vi "encoder_test_3mode_2motor_v4.vi"() -> ()   [LabVIEW 2014]
uses:
  <vilib>/rvi/FXPMathLib/FxpSinAndCos/subVIs/nifxpmath_SinAndCos_SimConfig.ctl
  <vilib>/rvi/Emulation/niFpgaGetClockAttributes.vi
  <vilib>/rvi/Emulation/niFpgaSctlEmulationGetInTimedLoop.vi
  <vilib>/rvi/Emulation/niFpgaEmulationReportErrorSimple.vi
  <vilib>/rvi/eio/common/nirviEmuTemplateMethod_errors.vi
  <vilib>/rvi/Emulation/niFpgaProcessEmulError.vi
  <vilib>/rvi/Emulation/niFpgaCriticalErrorInLSC.vi
  <vilib>/rvi/FXPMathLib/FxpSinAndCos/simVIs/DllFxpSinAndCosTemp_sub.vi
  <vilib>/rvi/interface/RandomDataEmulation/nirviRandomDataMultiElementFPGAFIFO.vi
  <instcachedir>/0/nirviRandomDataMultiElementFPGAFIFO_AD0CFC12EF974623A9C2E4184BC062B2.lvgen/nirviRandomDataMultiElementFPGAFIFO_AD0CFC12EF974623A9C2E4184BC062B2_020.vi
  <vilib>/rvi/interface/RandomDataEmulation/niFpgaRandomDataHandleErrors.vi
  <vilib>/eio/EIONode/EIONode.xnode
  <vilib>/rvi/FXPMathLib/FxpMul/XNode/nifxpmath_Multiplier.xnode
  <vilib>/rvi/FXPMathLib/FxpSinAndCos/XNode/nifxpmath_SinAndCos.xnode
  <vilib>/rvi/Analysis/measure/butterworth/XNode/niFpgaButterworthFilter.xnode
  <vilib>/rvi/FXPMathLib/FxpSub/XNode/nifxpmath_Sub.xnode
  <vilib>/rvi/FXPMathLib/FxpAdd/XNode/nifxpmath_Add.xnode
  <vilib>/rvi/DataTransferAndStorage/Container/XNode/niFpgaContainer.xnode
  <vilib>/rvi/interface/RandomDataEmulation/nirviRandomDataFpgaMultiElementTemplate.vi
  <vilib>/rvi/FXPMathLib/sim/FxpSim.dll
panel:
  in  "mt0_y":u32
  out "Dyr_sin_dd":fxp<+/-,64,25>
  out "Dyr_sin_d":fxp<+/-,64,16>
  out "Dyr_sin":fxp<+/-,30,11>
  in  "Sin offset_y":fxp<+/-,29,10>
  out "Sin omega_y":fxp<+/-,41,8>
  in  "Sin magnitude_y":fxp<+/-,11,8>
  in  "Sin frequency_y (Hz)":fxp<+/-,21,5>
  out "Dyr_ramp":fxp<+/-,32,7>
  out "Time now_y (s)":fxp<+,52,14>
  out "Dyr_slope":fxp<+/-,32,10>
  in  "Dyr_time":fxp<+/-,32,10>
  in  "Dyr_end":fxp<+/-,32,7>
  out "Dy_i":fxp<+/-,32,10>
  out "Dyr":fxp<+/-,32,7>
  in  "Direction_y":bool
  in  "Command type_y":i16(ring) items=["Step", "Ramp", "Sine"]
  out "Dy_error":fxp<+/-,24,8>
  out "Fmr_y":fxp<+/-,32,10>
  in  "Ki_y":fxp<+/-,20,6>
  in  "Dy_tolorence":fxp<+/-,18,1>
  in  "Kd_y":fxp<+/-,20,8>
  in  "Kp_y":fxp<+/-,20,8>
  in  "scaled coefficients_Dy_dd":i32[](array[numeric])=[780119100, 146811362]
  out "Dy_dd":fxp<+/-,36,10>
  out "va_y":fxp<+/-,38,8>
  out "vb_y":fxp<+/-,38,8>
  out "vd_y":fxp<+/-,20,5>
  out "vq_y":fxp<+/-,20,5> format="%.57g"
  in  "Stop motor_y":bool
  out "Dy_d (mm/s)":fxp<+/-,33,9>
  out "omega_y (rad/s)":fxp<+/-,32,7>
  in  "Velocity Estimation_y":i16(ring) items=["M_avg method", "M method", "T method"]
  out "Dy_d (T)":fxp<+/-,32,8>
  out "mt_y":u32
  out "omega_y (T)":fxp<+/-,32,7>
  out "omega_y (M)":fxp<+/-,32,7>
  out "Dy_d (M)":fxp<+/-,32,8>
  in  "Dy_d_M_Tc (mSec)":u32 format="%#_6f"
  out "omega_y(M_avg)":fxp<+/-,32,7>
  out "Dy_d (M_avg)":fxp<+,32,8>
  in  "Dy_d_M_avg_Tc (uSec)":u32
  out "rad_y(NrTheta)":fxp<+/-,33,18>
  out "Dy (mm)":fxp<+/-,22,7>
  out "Encoder Position_y":i32
  in  "Encoder Reset_y":bool
  out "omega_p (M_avg)":fxp<+/-,32,7>
  out "Dp_d (M_avg)":fxp<+/-,32,8>
  in  "Dp_d_M_avg_Tc (uSec)":u32 caption="D_d_M_avg_Tc (uSec)"
  out "omega_p (M)":fxp<+/-,32,7>
  out "Dp_d (M)":fxp<+/-,32,8>
  in  "Dp_d_M_Tc (mSec)":u32 format="%#_6f"
  out "Dp_d (T)":fxp<+/-,32,8>
  out "omega_p(T)":fxp<+/-,32,7>
  in  "Velocity Estimation_p":i16(ring) items=["M_avg method", "M method", "T method"]
  out "Dpr_ramp":fxp<+/-,64,30>
  out "Dpr_slope":fxp<+/-,32,10>
  in  "Dpr_time":fxp<+/-,32,10>
  out "Dpr_sin":fxp<+/-,30,11>
  out "Dpr_sin_d":fxp<+/-,64,16>
  out "Dpr_sin_dd":fxp<+/-,64,25>
  out "Sin omega_p":fxp<+/-,41,8>
  in  "Sin offset_p":fxp<+/-,27,10>
  in  "Sin magnitude_p":fxp<+/-,11,8>
  in  "Sin frequency_p (Hz)":fxp<+/-,21,5>
  out "Time now_p (s)":fxp<+,52,14>
  out "Dpr":fxp<+/-,32,7>
  in  "Dpr_end":fxp<+/-,22,7>
  in  "Command type_p":i16(ring) items=["Step", "Ramp", "Sine"]
  out "Dp_i":fxp<+/-,32,10>
  in  "Dp_tolorence":fxp<+/-,18,1>
  in  "Ki_p":fxp<+/-,20,6>
  out "Dp_error":fxp<+/-,24,8>
  in  "Direction_p":bool
  out "Fmr_p":fxp<+/-,32,10>
  in  "Kd_p":fxp<+/-,20,8>
  in  "Kp_p":fxp<+/-,20,12>
  in  "scaled coefficients_Dp_dd":i32[](array[numeric])=[780119100, 146811362]
  out "Dp_dd":fxp<+/-,36,10>
  in  "Ini coe.":bool
  out "va_p":fxp<+/-,38,8>
  out "vb_p":fxp<+/-,38,8>
  in  "Stop motor_p":bool
  out "vq_p":fxp<+/-,20,5> format="%.57g"
  out "vd_p":fxp<+/-,20,5>
  out "Dp_d (mm/s)":fxp<+/-,32,8>
  out "mt_p":u32
  out "omega_p (rad/s)":fxp<+/-,32,7>
  in  "mt0_p":u32
  out "Dp (mm)":fxp<+/-,22,7>
  out "rad_p(NrTheta)":fxp<+/-,33,18>
  out "Encoder Position_p":i32
  in  "Encoder Reset_p":bool
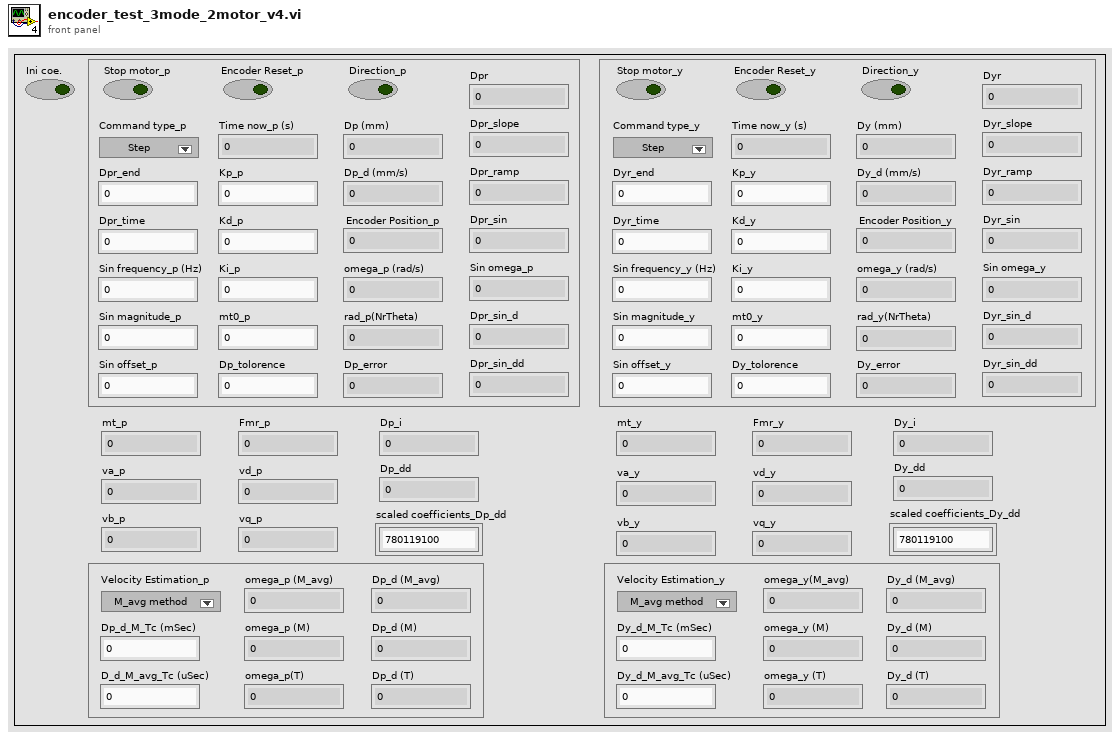
[diagram p1: front panel]
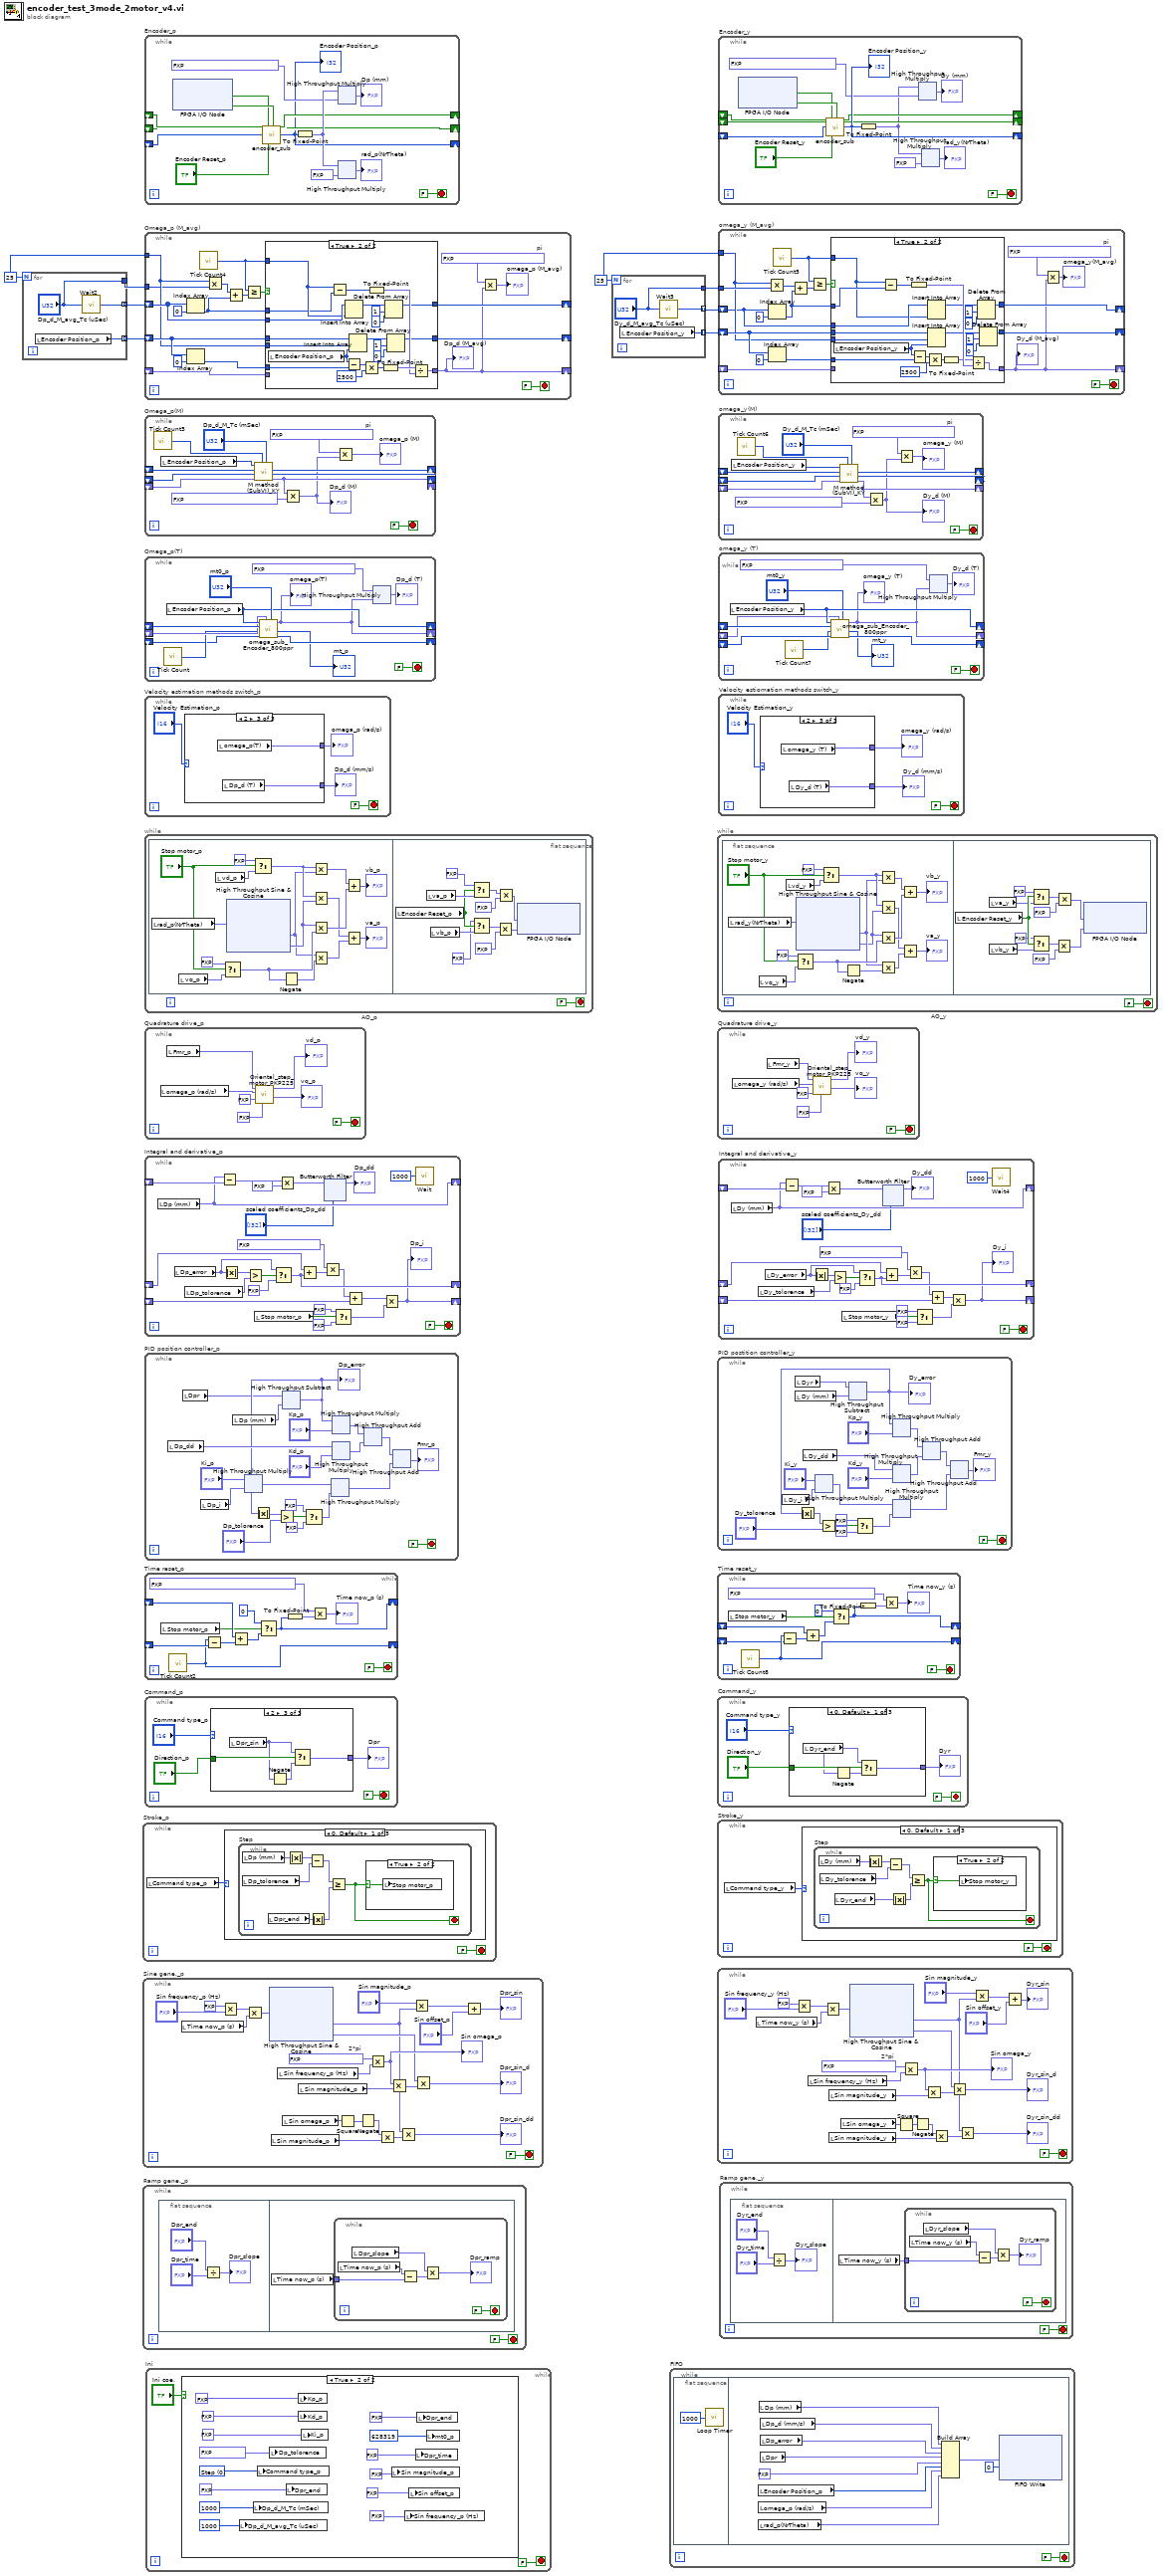
[diagram p0: block diagram]
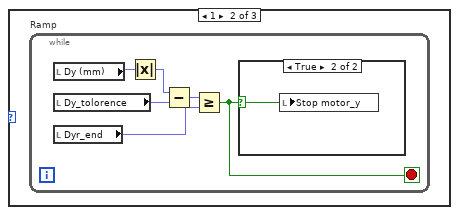
[diagram p3: hidden frame]
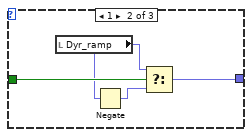
[diagram p6: hidden frame]
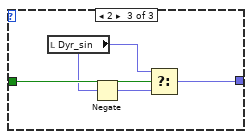
[diagram p7: hidden frame]
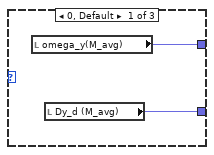
[diagram p8: hidden frame]
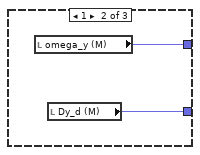
[diagram p9: hidden frame]
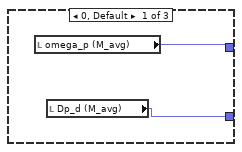
[diagram p12: hidden frame]
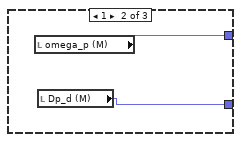
[diagram p13: hidden frame]
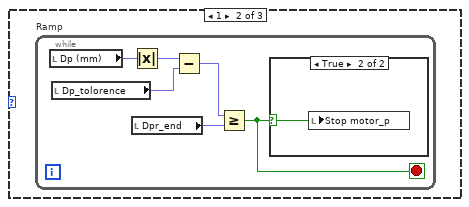
[diagram p15: hidden frame]
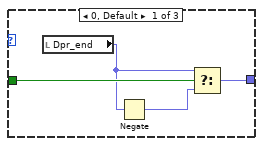
[diagram p18: hidden frame]
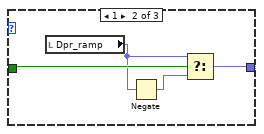
[diagram p19: hidden frame]
diagram:
  w4 = 25
  w8 = 25
  n1 = for {
    N: w8 -> [_]
    tunnel: ["Dp_d_M_avg_Tc (uSec)"] -> w5
    tunnel: [w10] -> w7 mode=indexing
    tunnel: [w9] -> w6 mode=indexing
    n2 = local read "Encoder Position_p"() -> (w9:i32)
    n3 = call "Wait2"("Count(uSec)"="Dp_d_M_avg_Tc (uSec)") -> ("Tick Count(uSec)"=w10:u32)
  }
  n4 = while "Stroke_p" {
    stop <- FALSE stop-if-true
    n5 = local read "Command type_p"() -> (w13:i16)
    n6 = case shown="0, Default" w13 {
      frame 0, Default {
        n7 = while "Step" {
          stop <- w14 stop-if-true
          n8 = local read "Dp_tolorence"() -> (w16:fxp<+/-,18,1>)
          n9 = local read "Dp (mm)"() -> (w18:fxp<+/-,22,7>)
          n10 = local read "Dpr_end"() -> (w20:fxp<+/-,22,7>)
          n11 = Absolute Value(x=w18) -> (abs(x)=w17:fxp<+,22,7>)
          n12 = Subtract(x=w17, y=w16) -> (x-y=w15:fxp<+/-,25,8>)
          n13 = Absolute Value(x=w20) -> (abs(x)=w19:fxp<+,22,7>)
          n14 = Greater Or Equal?(x=w15, y=w19) -> (x >= y?=w14:bool)
          n15 = case shown="True" w14 {
            selector: w14 -> [_ w21]
            frame False {
            }
            frame True {
              n16 = local write "Stop motor_p"(w21) -> ()
            }
          }
        }
      }
      frame 1 {
        n17 = while "Ramp" {
          stop <- w22 stop-if-true
          n18 = local read "Dp (mm)"() -> (w24:fxp<+/-,22,7>)
          n19 = local read "Dp_tolorence"() -> (w26:fxp<+/-,18,1>)
          n20 = Absolute Value(x=w24) -> (abs(x)=w25:fxp<+,22,7>)
          n21 = local read "Dpr_end"() -> (w23:fxp<+/-,22,7>)
          n22 = Subtract(x=w25, y=w26) -> (x-y=w27:fxp<+/-,25,8>)
          n23 = Greater Or Equal?(x=w27, y=w23) -> (x >= y?=w22:bool)
          n24 = case shown="True" w22 {
            selector: w22 -> [_ w28]
            frame False {
            }
            frame True {
              n25 = local write "Stop motor_p"(w28) -> ()
            }
          }
        }
      }
      frame 2 {
      }
    }
  }
  n26 = while "Sine gene._p" {
    stop <- FALSE stop-if-true
    w46 = fxp<+,20,3> 6.2831878662109375  # 2*pi
    n27 = local read "Time now_p (s)"() -> (w49:fxp<+,52,14>)
    n28 = Multiply(x=fxp<+,1,2> 2.0, y="Sin frequency_p (Hz)") -> (x*y=w50:fxp<+/-,21,6>)
    n29 = Multiply(x=w50, y=w49) -> (x*y=w30:fxp<+/-,64,20>)
    n30 = xnode "High Throughput Sine & Cosine"("x (pi)"=w30) -> ("sin(x)"=w34:fxp<+/-,18,2>, "cos(x)"=w41:fxp<+/-,18,2>)
    n31 = local read "Sin magnitude_p"() -> (w36:fxp<+/-,11,8>)
    n32 = local read "Sin frequency_p (Hz)"() -> (w45:fxp<+/-,21,5>)
    n33 = local read "Sin omega_p"() -> (w37:fxp<+/-,41,8>)
    n34 = local read "Sin magnitude_p"() -> (w40:fxp<+/-,11,8>)
    n35 = Square(x=w37) -> (x^2=w38:fxp<+,64,14>)
    n36 = Negate(x=w38) -> (-x=w35:fxp<+/-,64,15>)
    n37 = Multiply(x=w46, y=w45) -> (x*y=w42:fxp<+/-,41,8>)
    "Sin omega_p" <- w42
    n38 = Multiply(x=w35, y=w36) -> (x*y=w39:fxp<+/-,64,23>)
    n39 = Multiply(x=w42, y=w40) -> (x*y=w47:fxp<+/-,51,15>)
    n40 = Multiply(x=w34, y=w39) -> (x*y=→"Dpr_sin_dd":fxp<+/-,64,25>)
    n41 = Multiply(x="Sin magnitude_p", y=w34) -> (x*y=w48:fxp<+/-,29,10>)
    n42 = Multiply(x=w41, y=w47) -> (x*y=→"Dpr_sin_d":fxp<+/-,64,16>)
    n43 = Add(x=w48, y="Sin offset_p") -> (x+y=→"Dpr_sin":fxp<+/-,30,11>)
  }
  n44 = while "Ramp gene._p" {
    stop <- FALSE stop-if-true
    n45 = flat-sequence {
      frame #0 {
        n46 = Divide(x="Dpr_end", y="Dpr_time") -> (x/y=→"Dpr_slope":fxp<+/-,55,30>)
      }
      frame #1 {
        n47 = local read "Time now_p (s)"() -> (w87:fxp<+,52,14>)
        n48 = while {
          tunnel: w87 -> [w93]
          stop <- FALSE stop-if-true
          n49 = local read "Time now_p (s)"() -> (w90:fxp<+,52,14>)
          n50 = local read "Dpr_slope"() -> (w91:fxp<+/-,32,10>)
          n51 = Subtract(x=w90, y=w93) -> (x-y=w92:fxp<+/-,53,15>)
          n52 = Multiply(x=w91, y=w92) -> (x*y=→"Dpr_ramp":fxp<+/-,64,24>)
        }
      }
    }
  }
  n53 = while "Encoder_p" {
    shift-right: [w100] -> _
    shift-left: _ -> [w102]
    shift-right: [w99] -> _
    shift-left: _ -> [w101]
    shift-right: [w97] -> _
    shift-left: _ -> [w98]
    stop <- FALSE stop-if-true
    n54 = xnode "FPGA I/O Node"() -> ("Mod4/DI3"=w107:bool, "Mod4/DI4"=w108:bool)  [unwired: 2 in, 2 out]
    n55 = call "encoder_sub.vi"("A_pre"=w102, "B_pre"=w101, "Encoder Position_pre"=w98, "A input"=w107, "Encoder Position Reset"="Encoder Reset_p", "B input"=w108) -> ("A"=w100:bool, "B"=w99:bool, "Encoder Position (Counts)"=w97:i32)  [unwired: 19 in]
    "Encoder Position_p" <- w97
    n56 = To Fixed-Point(number=w97) -> (fixed-point=w105:fxp<+/-,32,32>)  [unwired: 1 in]
    n57 = xnode ("High Throughput Multiply")("x"=w105, "y"=fxp<+/-,24,0> 0.002499997615814209) -> ("x*y"=→"Dp (mm)":fxp<+/-,56,32>)
    n58 = xnode ("High Throughput Multiply")("x"=w105, "y"=fxp<+/-,24,0> 0.125) -> ("x*y"=→"rad_p(NrTheta)":fxp<+/-,56,32>)
  }
  n59 = while "Omega_p (M_avg)" {
    tunnel: w8 -> [w120]
    shift-right: [w113] -> _
    shift-left: w7 -> [w124]
    shift-right: [w112] -> _
    shift-left: _ -> [w115]
    shift-right: [w114] -> _
    shift-left: w6 -> [w123]
    tunnel: w5 -> [w117]
    stop <- FALSE stop-if-true
    w111 = fxp<+/-,27,3> 3.1415926218032837  # pi
    n60 = Index Array(array=w124, index=0) -> (element=w118:u32)
    n61 = Index Array(array=w123, index=0) -> (element=w119:i32)
    n62 = call "Tick Count4"() -> ("Tick Count(uSec)"=w121:u32)
    n63 = Multiply(x=w120, y=w117) -> (x*y=w125:u32)
    n64 = Add(x=w125, y=w118) -> (x+y=w122:u32)
    n65 = Greater Or Equal?(x=w121, y=w122) -> (x >= y?=w116:bool)
    n66 = case shown="True" w116 {
      tunnel: w124 -> [w130 w147]
      tunnel: w123 -> [w129 w146]
      tunnel: w121 -> [_ w139]
      tunnel: w120 -> [_ w145]
      tunnel: w119 -> [_ w143]
      tunnel: w118 -> [_ w138]
      tunnel: w115 -> [w128 _]
      tunnel: [w129 w133] -> w114
      tunnel: [w130 w132] -> w113
      tunnel: [w128 w131] -> w112
      frame False {
      }
      frame True {
        n67 = local read "Encoder Position_p"() -> (w144:i32)
        n68 = Subtract(x=w139, y=w138) -> (x-y=w136:u32)
        n69 = Insert Into Array(array=w147, new element=w139) -> (w148:u32[])  [unwired: 1 in]
        n70 = Subtract(x=w144, y=w143) -> (x-y=w142:i32)
        n71 = Insert Into Array(array=w146, index=w145, new element=w144) -> (w149:i32[])
        n72 = Multiply(x=w142, y=2500) -> (x*y=w140:i32)
        n73 = To Fixed-Point(number=w136) -> (fixed-point=w134:fxp<+,32,32>)  [unwired: 1 in]
        n74 = To Fixed-Point(number=w140) -> (fixed-point=w135:fxp<+/-,32,32>)  [unwired: 1 in]
        n75 = Delete From Array(array=w148, length=1, index=0) -> (array with subset deleted=w132:u32[])  [unwired: 1 out]
        n76 = Delete From Array(array=w149, length=1, index=0) -> (array with subset deleted=w133:i32[])  [unwired: 1 out]
        n77 = Divide(x=w135, y=w134) -> (x/y=w131:fxp<+/-,64,32>)
      }
    }
    "Dp_d (M_avg)" <- w112
    n78 = Multiply(x=w111, y=w112) -> (x*y=→"omega_p (M_avg)":fxp<+/-,64,35>)
  }
  n79 = while "Omega_p(M)" {
    shift-right: [w164] -> _
    shift-left: _ -> [w165]
    shift-right: [w160] -> _
    shift-left: _ -> [w161]
    shift-right: [w158] -> _
    shift-left: _ -> [w159]
    stop <- FALSE stop-if-true
    w155 = fxp<+/-,27,3> 3.1415926218032837  # pi
    n80 = call "Tick Count3"() -> ("Tick Count(mSec)"=w163:u32)
    n81 = local read "Encoder Position_p"() -> (w166:i32)
    n82 = call "M method (SubVI)_KY.vi"("Tc (mSec)"="Dp_d_M_Tc (mSec)", "Tick Count (mSec)"=w163, "Encoder velocity_pre (pulse/s)"=w159, "Shift Register in 2"=w161, "Shift Register in 1"=w165, "Encoder pulses"=w166) -> ("Encoder velocity (pulse/s)"=w158:fxp<+/-,64,32>, "Shift Register out 2"=w160:i32, "Shift Register out 1"=w164:u32)  [unwired: 3 in]
    n83 = Multiply(x=w158, y=fxp<+/-,20,-5> 0.002499997615814209) -> (x*y=w156:fxp<+/-,64,27>)
    "Dp_d (M)" <- w156
    n84 = Multiply(x=w155, y=w156) -> (x*y=→"omega_p (M)":fxp<+/-,64,30>)
  }
  n85 = while "Omega_p(T)" {
    shift-right: [w176] -> _
    shift-left: _ -> [w177]
    shift-right: [w169] -> _
    shift-left: _ -> [w175]
    shift-right: [w172] -> _
    shift-left: _ -> [w173]
    stop <- FALSE stop-if-true
    n86 = call "Tick Count"() -> ("Tick Count(Ticks)"=w174:u32)
    n87 = local read "Encoder Position_p"() -> (w176:i32)
    n88 = call "omega_sub_Encoder_800ppr.vi"("mt0"="mt0_p", "omega_pre"=w175, "ticks_m_pre"=w173, "ticks"=w174, "count_pre"=w177, "count"=w176) -> ("ticks_m"=w172:u32, "mt"=→"mt_p":u32, "omega"=w169:fxp<+/-,20,9>)  [unwired: 3 in]
    "omega_p(T)" <- w169
    n89 = xnode ("High Throughput Multiply")("x"=fxp<+/-,26,1> 0.3183099031448364, "y"=w169) -> ("x*y"=→"Dp_d (T)":fxp<+/-,46,10>)
  }
  n90 = while "Velocity estimation methods switch_p" {
    stop <- FALSE stop-if-true
    n91 = case shown="2" "Velocity Estimation_p" {
      tunnel: [w184 w186 w188] -> w181
      tunnel: [w183 w185 w187] -> w180
      frame 0, Default {
        n92 = local read "omega_p (M_avg)"() -> (w184:fxp<+/-,32,7>)
        n93 = local read "Dp_d (M_avg)"() -> (w183:fxp<+/-,32,8>)
      }
      frame 1 {
        n94 = local read "omega_p (M)"() -> (w186:fxp<+/-,32,7>)
        n95 = local read "Dp_d (M)"() -> (w185:fxp<+/-,32,8>)
      }
      frame 2 {
        n96 = local read "omega_p(T)"() -> (w188:fxp<+/-,32,7>)
        n97 = local read "Dp_d (T)"() -> (w187:fxp<+/-,32,8>)
      }
    }
    "Dp_d (mm/s)" <- w180
    "omega_p (rad/s)" <- w181
  }
  n98 = while "AO_p" {
    stop <- FALSE stop-if-true
    n99 = flat-sequence {
      frame #0 {
        n100 = local read "rad_p(NrTheta)"() -> (w205:fxp<+/-,33,18>)
        n101 = local read "vq_p"() -> (w203:fxp<+/-,20,5>)
        n102 = local read "vd_p"() -> (w204:fxp<+/-,20,5>)
        n103 = Select(t=fxp<+,20,5> 0.0, s="Stop motor_p", f=w203) -> (s? t:f=w200:fxp<+/-,21,6>)
        n104 = xnode "High Throughput Sine & Cosine"("x (pi)"=w205) -> ("sin(x)"=w196:fxp<+/-,17,2>, "cos(x)"=w198:fxp<+/-,17,2>)
        n105 = Select(t=fxp<+,20,5> 0.0, s="Stop motor_p", f=w204) -> (s? t:f=w197:fxp<+/-,21,6>)
        n106 = Negate(x=w200) -> (-x=w199:fxp<+/-,21,6>)
        n107 = Multiply(x=w197, y=w196) -> (x*y=w195:fxp<+/-,37,7>)
        n108 = Multiply(x=w197, y=w198) -> (x*y=w193:fxp<+/-,37,7>)
        n109 = Multiply(x=w198, y=w200) -> (x*y=w194:fxp<+/-,37,7>)
        n110 = Multiply(x=w196, y=w199) -> (x*y=w192:fxp<+/-,37,7>)
        n111 = Add(x=w195, y=w194) -> (x+y=→"vb_p":fxp<+/-,38,8>)
        n112 = Add(x=w193, y=w192) -> (x+y=→"va_p":fxp<+/-,38,8>)
      }
      frame #1 {
        n113 = local read "Encoder Reset_p"() -> (w239:bool)
        n114 = local read "va_p"() -> (w241:fxp<+/-,38,8>)
        n115 = local read "vb_p"() -> (w240:fxp<+/-,38,8>)
        n116 = Select(t=fxp<+/-,20,5> 5.0 ("y"), s=w239, f=w241) -> (s? t:f=w242:fxp<+/-,38,8>)
        n117 = Select(t=fxp<+/-,20,5> 0.0 ("y"), s=w239, f=w240) -> (s? t:f=w243:fxp<+/-,38,8>)
        n118 = Multiply(x=w243, y=fxp<+/-,20,5> -0.5) -> (x*y=w247:fxp<+/-,57,12>)
        n119 = Multiply(x=w242, y=fxp<+/-,20,5> -0.5) -> (x*y=w246:fxp<+/-,57,12>)
        n120 = xnode "FPGA I/O Node"("Mod8/AO0"=w246, "Mod8/AO1"=w247) -> ()  [unwired: 2 in, 2 out]
      }
    }
  }
  n121 = while "Quadrature drive_p" {
    stop <- FALSE stop-if-true
    n122 = local read "omega_p (rad/s)"() -> (w250:fxp<+/-,32,7>)
    n123 = local read "Fmr_p"() -> (w248:fxp<+/-,32,10>)
    n124 = call "Oriental_step_motor_PKP225.vi"("F_Threshold"=fxp<+,12,12> 10.0, "dFmr"=fxp<+/-,25,15> 0.0, "omega"=w250, "Fmr"=w248) -> ("vq_F"=→"vq_p":fxp<+/-,20,5>, "vd_F"=→"vd_p":fxp<+/-,20,5>)  [unwired: 6 in]
  }
  n125 = while "Integral and derivative_p" {
    shift-right: [w275] -> _
    shift-left: _ -> [w279]
    shift-right: [w265] -> _
    shift-left: _ -> [w266]
    shift-right: [w255] -> _
    shift-left: _ -> [w259]
    stop <- FALSE stop-if-true
    n126 = local read "Dp (mm)"() -> (w275:fxp<+/-,22,7>)
    n127 = local read "Dp_error"() -> (w267:fxp<+/-,24,8>)
    n128 = local read "Dp_tolorence"() -> (w270:fxp<+/-,18,1>)
    n129 = Subtract(x=w275, y=w279) -> (x-y=w278:fxp<+/-,23,8>)
    n130 = Absolute Value(x=w267) -> (abs(x)=w271:fxp<+,24,8>)
    n131 = Greater?(x=w271, y=w270) -> (0:w269:bool)
    n132 = local read "Stop motor_p"() -> (w262:bool)
    n133 = Select(t=w267, s=w269, f=fxp<+,24,11> 0.0) -> (s? t:f=w265:fxp<+/-,28,12>)
    n134 = Multiply(x=w278, y=fxp<+/-,33,13> 1000.0) -> (x*y=w276:fxp<+/-,55,20>)
    n135 = Add(x=w266, y=w265) -> (x+y=w264:fxp<+/-,29,13>)
    n136 = Multiply(x=fxp<+/-,30,12> 0.000499725341796875, y=w264) -> (x*y=w258:fxp<+/-,58,24>)
    n137 = xnode "Butterworth Filter"("input data"=w276, "scaled coefficients"="scaled coefficients_Dp_dd") -> ("output data"=→"Dp_dd":fxp<+/-,36,24>)  [unwired: 1 in]
    n138 = Select(t=fxp<+,1,1> 0.0, s=w262, f=fxp<+,1,1> 1.0) -> (s? t:f=w256:fxp<+,1,1>)
    n139 = Add(x=w258, y=w259) -> (x+y=w257:fxp<+/-,32,16>)
    n140 = Multiply(x=w257, y=w256) -> (x*y=w255:fxp<+/-,32,16>)
    "Dp_i" <- w255
    n141 = call "Wait"("Count(uSec)"=u32 1000) -> ()  [unwired: 1 out]
  }
  n142 = while "PID position controller_p" {
    stop <- FALSE stop-if-true
    n143 = local read "Dp_dd"() -> (w305:fxp<+/-,36,10>)
    n144 = local read "Dpr"() -> (w289:fxp<+/-,32,7>)
    n145 = local read "Dp_i"() -> (w300:fxp<+/-,32,10>)
    n146 = local read "Dp (mm)"() -> (w309:fxp<+/-,22,7>)
    n147 = xnode ("High Throughput Multiply")("x"="Ki_p", "y"=w300) -> ("x*y"=w294:fxp<+/-,52,16>)
    n148 = xnode "High Throughput Subtract"("x"=w289, "y"=w309) -> ("x-y"=w298:fxp<+/-,33,8>)
    "Dp_error" <- w298
    n149 = Absolute Value(x=w298) -> (abs(x)=w299:fxp<+,33,8>)
    n150 = Greater?(x=w299, y="Dp_tolorence") -> (0:w297:bool)
    n151 = Select(t=fxp<+,10,2> 1.0, s=w297, f=fxp<+,10,2> 0.0) -> (s? t:f=w293:fxp<+,10,2>)
    n152 = xnode ("High Throughput Multiply")("x"=w294, "y"=w293) -> ("x*y"=w290:fxp<+/-,62,18>)
    n153 = xnode ("High Throughput Multiply")("x"=w298, "y"="Kp_p") -> ("x*y"=w307:fxp<+/-,53,20>)
    n154 = xnode ("High Throughput Multiply")("x"=w305, "y"="Kd_p") -> ("x*y"=w306:fxp<+/-,56,18>)
    n155 = xnode ("High Throughput Add")("x"=w307, "y"=w306) -> ("x+y"=w291:fxp<+/-,59,21>)
    n156 = xnode ("High Throughput Add")("x"=w291, "y"=w290) -> ("x+y"=→"Fmr_p":fxp<+/-,64,22>)
  }
  n157 = while "Time reset_p" {
    shift-right: [w313] -> _
    shift-left: _ -> [w320]
    shift-right: [w315] -> _
    shift-left: _ -> [w316]
    stop <- FALSE stop-if-true
    n158 = local read "Stop motor_p"() -> (w318:bool)
    n159 = call "Tick Count2"() -> ("Tick Count(uSec)"=w315:u32)
    n160 = Subtract(x=w315, y=w316) -> (x-y=w321:u32)
    n161 = Add(x=w320, y=w321) -> (x+y=w319:u32)
    n162 = Select(t=u32 0, s=w318, f=w319) -> (s? t:f=w313:u32)
    n163 = To Fixed-Point(number=w313) -> (fixed-point=w312:fxp<+,32,32>)  [unwired: 1 in]
    n164 = Multiply(x=fxp<+,20,-18> 1.0000003385357559e-06, y=w312) -> (x*y=→"Time now_p (s)":fxp<+,52,14>)
  }
  n165 = while "Command_p" {
    stop <- FALSE stop-if-true
    n166 = case shown="2" "Command type_p" {
      tunnel: [w326 w330 w334] -> w324
      tunnel: "Direction_p" -> [w329 w333 w337]
      frame 0, Default {
        n167 = local read "Dpr_end"() -> (w328:fxp<+/-,22,7>)
        n168 = Negate(x=w328) -> (-x=w327:fxp<+/-,23,8>)
        n169 = Select(t=w328, s=w329, f=w327) -> (s? t:f=w326:fxp<+/-,23,8>)
      }
      frame 1 {
        n170 = local read "Dpr_ramp"() -> (w331:fxp<+/-,64,30>)
        n171 = Negate(x=w331) -> (-x=w332:fxp<+/-,64,31>)
        n172 = Select(t=w331, s=w333, f=w332) -> (s? t:f=w330:fxp<+/-,64,31>)
      }
      frame 2 {
        n173 = local read "Dpr_sin"() -> (w335:fxp<+/-,30,11>)
        n174 = Negate(x=w335) -> (-x=w336:fxp<+/-,29,10>)
        n175 = Select(t=w335, s=w337, f=w336) -> (s? t:f=w334:fxp<+/-,30,11>)
      }
    }
    "Dpr" <- w324
  }
  n176 = while "Ini" {
    stop <- FALSE stop-if-true
    n177 = case shown="True" "Ini coe." {
      frame False {
      }
      frame True {
        w347 = i16 0 items=["Step", "Ramp", "Sine"] ("Command type")
        n178 = local write "Dp_d_M_avg_Tc (uSec)"(u32 1000 ("D_d_M_avg_Tc (uSec)")) -> ()
        n179 = local write "Dp_d_M_Tc (mSec)"(u32 1000 ("D_d_M_Tc (uSec)")) -> ()
        n180 = local write "Command type_p"(w347) -> ()
        n181 = local write "Dp_tolorence"(fxp<+/-,14,3> 0.009765625 ("D_tolorence")) -> ()
        n182 = local write "Dpr_end"(fxp<+/-,16,11> 20.0 ("Dr_end")) -> ()
        n183 = local write "Kp_p"(fxp<+/-,20,12> 10.0 ("Kp")) -> ()
        n184 = local write "Kd_p"(fxp<+/-,20,8> 2.0 ("Kd")) -> ()
        n185 = local write "Ki_p"(fxp<+/-,20,6> 8.0 ("D_i")) -> ()
        n186 = local write "Sin magnitude_p"(fxp<+/-,11,8> 20.0 ("Sin magnitude")) -> ()
        n187 = local write "Sin frequency_p (Hz)"(fxp<+/-,21,5> 0.5 ("Sin wave frequency (Hz)")) -> ()
        n188 = local write "Sin offset_p"(fxp<+/-,27,10> 0.0 ("Sin offset")) -> ()
        n189 = local write "Dpr_time"(fxp<+/-,16,11> 5.0 ("Dr_time")) -> ()
        n190 = local write "Dpr_end"(fxp<+/-,11,7> 20.0 ("Fmr")) -> ()
        n191 = local write "mt0_p"(u32 628319 ("mt0")) -> ()
      }
    }
  }
  n192 = for {
    N: w4 -> [_]
    tunnel: ["Dy_d_M_avg_Tc (uSec)"] -> w3
    tunnel: [w355] -> w1 mode=indexing
    tunnel: [w354] -> w2 mode=indexing
    n193 = local read "Encoder Position_y"() -> (w354:i32)
    n194 = call "Wait3"("Count(uSec)"="Dy_d_M_avg_Tc (uSec)") -> ("Tick Count(uSec)"=w355:u32)
  }
  n195 = while "FIFO" {
    stop <- FALSE stop-if-true
    n196 = flat-sequence {
      frame #0 {
        n197 = call "Loop Timer"("Count(uSec)"=u32 1000) -> ()  [unwired: 1 out]
      }
      frame #1 {
        n198 = local read "Encoder Position_p"() -> (w362:i32)
        n199 = local read "omega_p (rad/s)"() -> (w361:fxp<+/-,32,7>)
        n200 = local read "rad_p(NrTheta)"() -> (w360:fxp<+/-,33,18>)
        n201 = local read "Dp (mm)"() -> (w366:fxp<+/-,22,7>)
        n202 = local read "Dp_d (mm/s)"() -> (w365:fxp<+/-,32,8>)
        n203 = local read "Dp_error"() -> (w364:fxp<+/-,24,8>)
        n204 = local read "Dpr"() -> (w363:fxp<+/-,32,7>)
        n205 = Build Array(w366, w365, w364, w363, fxp<+/-,64,32> 0.0 ("element"), w362, w361, w360) -> (w367:fxp<+/-,64,32>[])
        n206 = xnode ("FIFO Write")("Element"=w367, "Timeout"=0) -> ()  [unwired: 1 in, 2 out]
      }
    }
  }
  n207 = while "AO_y" {
    stop <- FALSE stop-if-true
    n208 = flat-sequence {
      frame #0 {
        n209 = local read "rad_y(NrTheta)"() -> (w381:fxp<+/-,33,18>)
        n210 = local read "vq_y"() -> (w384:fxp<+/-,20,5>)
        n211 = local read "vd_y"() -> (w383:fxp<+/-,20,5>)
        n212 = xnode "High Throughput Sine & Cosine"("x (pi)"=w381) -> ("sin(x)"=w377:fxp<+/-,17,2>, "cos(x)"=w376:fxp<+/-,17,2>)
        n213 = Select(t=fxp<+,20,5> 0.0, s="Stop motor_y", f=w384) -> (s? t:f=w379:fxp<+/-,21,6>)
        n214 = Select(t=fxp<+/-,20,5> 0.0, s="Stop motor_y", f=w383) -> (s? t:f=w378:fxp<+/-,20,5>)
        n215 = Negate(x=w379) -> (-x=w380:fxp<+/-,21,6>)
        n216 = Multiply(x=w378, y=w377) -> (x*y=w375:fxp<+/-,37,7>)
        n217 = Multiply(x=w378, y=w376) -> (x*y=w373:fxp<+/-,37,7>)
        n218 = Multiply(x=w376, y=w379) -> (x*y=w374:fxp<+/-,37,7>)
        n219 = Multiply(x=w377, y=w380) -> (x*y=w372:fxp<+/-,37,7>)
        n220 = Add(x=w375, y=w374) -> (x+y=→"vb_y":fxp<+/-,38,8>)
        n221 = Add(x=w373, y=w372) -> (x+y=→"va_y":fxp<+/-,38,8>)
      }
      frame #1 {
        n222 = local read "Encoder Reset_y"() -> (w427:bool)
        n223 = local read "va_y"() -> (w426:fxp<+/-,38,8>)
        n224 = local read "vb_y"() -> (w425:fxp<+/-,38,8>)
        n225 = Select(t=fxp<+/-,20,5> 5.0, s=w427, f=w426) -> (s? t:f=w422:fxp<+/-,38,8>)
        n226 = Select(t=fxp<+/-,20,5> 0.0, s=w427, f=w425) -> (s? t:f=w421:fxp<+/-,38,8>)
        n227 = Multiply(x=w421, y=fxp<+/-,20,5> -0.5) -> (x*y=w417:fxp<+/-,57,12>)
        n228 = Multiply(x=w422, y=fxp<+/-,20,5> -0.5) -> (x*y=w418:fxp<+/-,57,12>)
        n229 = xnode "FPGA I/O Node"("Mod8/AO2"=w418, "Mod8/AO3"=w417) -> ()  [unwired: 2 in, 2 out]
      }
    }
  }
  n230 = while "Quadrature drive_y" {
    stop <- FALSE stop-if-true
    n231 = local read "omega_y (rad/s)"() -> (w434:fxp<+/-,32,7>)
    n232 = local read "Fmr_y"() -> (w429:fxp<+/-,32,10>)
    n233 = call "Oriental_step_motor_PKP225.vi"("F_Threshold"=fxp<+,12,12> 10.0, "dFmr"=fxp<+/-,25,15> 0.0, "omega"=w434, "Fmr"=w429) -> ("vq_F"=→"vq_y":fxp<+/-,20,5>, "vd_F"=→"vd_y":fxp<+/-,20,5>)  [unwired: 6 in]
  }
  n234 = while "PID postition controller_y" {
    stop <- FALSE stop-if-true
    n235 = local read "Dy_i"() -> (w436:fxp<+/-,32,10>)
    n236 = local read "Dyr"() -> (w437:fxp<+/-,32,7>)
    n237 = local read "Dy (mm)"() -> (w446:fxp<+/-,22,7>)
    n238 = local read "Dy_dd"() -> (w447:fxp<+/-,36,10>)
    n239 = xnode "High Throughput Multiply"("x"="Ki_y", "y"=w436) -> ("x*y"=w445:fxp<+/-,52,16>)
    n240 = xnode "High Throughput Subtract"("x"=w437, "y"=w446) -> ("x-y"=w438:fxp<+/-,33,8>)
    "Dy_error" <- w438
    n241 = Absolute Value(x=w438) -> (abs(x)=w439:fxp<+,33,8>)
    n242 = Greater?(x=w439, y="Dy_tolorence") -> (0:w450:bool)
    n243 = Select(t=fxp<+,1,1> 1.0, s=w450, f=fxp<+,1,1> 0.0) -> (s? t:f=w453:fxp<+,1,1>)
    n244 = xnode "High Throughput Multiply"("x"=w438, "y"="Kp_y") -> ("x*y"=w444:fxp<+/-,53,16>)
    n245 = xnode "High Throughput Multiply"("x"=w447, "y"="Kd_y") -> ("x*y"=w443:fxp<+/-,56,18>)
    n246 = xnode "High Throughput Multiply"("x"=w445, "y"=w453) -> ("x*y"=w441:fxp<+/-,52,16>)
    n247 = xnode "High Throughput Add"("x"=w444, "y"=w443) -> ("x+y"=w442:fxp<+/-,57,19>)
    n248 = xnode "High Throughput Add"("x"=w442, "y"=w441) -> ("x+y"=→"Fmr_y":fxp<+/-,58,20>)
  }
  n249 = while "Time reset_y" {
    shift-right: [w462] -> _
    shift-left: _ -> [w461]
    shift-right: [w460] -> _
    shift-left: _ -> [w463]
    stop <- FALSE stop-if-true
    n250 = local read "Stop motor_y"() -> (w467:bool)
    n251 = call "Tick Count8"() -> ("Tick Count(uSec)"=w462:u32)
    n252 = Subtract(x=w462, y=w461) -> (x-y=w466:u32)
    n253 = Add(x=w463, y=w466) -> (x+y=w464:u32)
    n254 = Select(t=u32 0, s=w467, f=w464) -> (s? t:f=w460:u32)
    n255 = To Fixed-Point(number=w460) -> (fixed-point=w459:fxp<+,32,32>)  [unwired: 1 in]
    n256 = Multiply(x=fxp<+,20,-18> 1.0000003385357559e-06, y=w459) -> (x*y=→"Time now_y (s)":fxp<+,52,14>)
  }
  n257 = while "Command_y" {
    stop <- FALSE stop-if-true
    n258 = case shown="0, Default" "Command type_y" {
      tunnel: "Direction_y" -> [w475 w479 w482]
      tunnel: [w474 w476 w483] -> w469
      frame 0, Default {
        n259 = local read "Dyr_end"() -> (w472:fxp<+/-,32,7>)
        n260 = Negate(x=w472) -> (-x=w473:fxp<+/-,33,8>)
        n261 = Select(t=w472, s=w475, f=w473) -> (s? t:f=w474:fxp<+/-,33,8>)
      }
      frame 1 {
        n262 = local read "Dyr_ramp"() -> (w477:fxp<+/-,32,7>)
        n263 = Negate(x=w477) -> (-x=w478:fxp<+/-,33,8>)
        n264 = Select(t=w477, s=w479, f=w478) -> (s? t:f=w476:fxp<+/-,33,8>)
      }
      frame 2 {
        n265 = local read "Dyr_sin"() -> (w480:fxp<+/-,30,11>)
        n266 = Negate(x=w480) -> (-x=w481:fxp<+/-,29,10>)
        n267 = Select(t=w480, s=w482, f=w481) -> (s? t:f=w483:fxp<+/-,30,11>)
      }
    }
    "Dyr" <- w469
  }
  n268 = while "Stroke_y" {
    stop <- FALSE stop-if-true
    n269 = local read "Command type_y"() -> (w485:i16)
    n270 = case shown="0, Default" w485 {
      frame 0, Default {
        n271 = while "Step" {
          stop <- w487 stop-if-true
          n272 = local read "Dy (mm)"() -> (w492:fxp<+/-,22,7>)
          n273 = local read "Dy_tolorence"() -> (w490:fxp<+/-,18,1>)
          n274 = local read "Dyr_end"() -> (w486:fxp<+/-,32,7>)
          n275 = Absolute Value(x=w492) -> (abs(x)=w491:fxp<+,22,7>)
          n276 = Subtract(x=w491, y=w490) -> (x-y=w489:fxp<+/-,25,8>)
          n277 = Absolute Value(x=w486) -> (abs(x)=w488:fxp<+,32,7>)
          n278 = Greater Or Equal?(x=w489, y=w488) -> (x >= y?=w487:bool)
          n279 = case shown="True" w487 {
            selector: w487 -> [_ w493]
            frame False {
            }
            frame True {
              n280 = local write "Stop motor_y"(w493) -> ()
            }
          }
        }
      }
      frame 1 {
        n281 = while "Ramp" {
          stop <- w494 stop-if-true
          n282 = local read "Dy (mm)"() -> (w498:fxp<+/-,22,7>)
          n283 = local read "Dy_tolorence"() -> (w497:fxp<+/-,18,1>)
          n284 = local read "Dyr_end"() -> (w495:fxp<+/-,32,7>)
          n285 = Absolute Value(x=w498) -> (abs(x)=w499:fxp<+,22,7>)
          n286 = Subtract(x=w499, y=w497) -> (x-y=w496:fxp<+/-,25,8>)
          n287 = Greater Or Equal?(x=w496, y=w495) -> (x >= y?=w494:bool)
          n288 = case shown="True" w494 {
            selector: w494 -> [_ w500]
            frame False {
            }
            frame True {
              n289 = local write "Stop motor_y"(w500) -> ()
            }
          }
        }
      }
      frame 2 {
      }
    }
  }
  n290 = while {
    stop <- FALSE stop-if-true
    w516 = fxp<+,20,3> 6.2831878662109375  # 2*pi
    n291 = local read "Time now_y (s)"() -> (w523:fxp<+,52,14>)
    n292 = Multiply(x=fxp<+,1,2> 2.0, y="Sin frequency_y (Hz)") -> (x*y=w522:fxp<+/-,21,6>)
    n293 = local read "Sin frequency_y (Hz)"() -> (w515:fxp<+/-,21,5>)
    n294 = Multiply(x=w522, y=w523) -> (x*y=w524:fxp<+/-,64,20>)
    n295 = local read "Sin magnitude_y"() -> (w514:fxp<+/-,11,8>)
    n296 = local read "Sin magnitude_y"() -> (w509:fxp<+/-,11,8>)
    n297 = local read "Sin omega_y"() -> (w510:fxp<+/-,41,8>)
    n298 = xnode "High Throughput Sine & Cosine"("x (pi)"=w524) -> ("sin(x)"=w507:fxp<+/-,18,2>, "cos(x)"=w511:fxp<+/-,18,2>)
    n299 = Square(x=w510) -> (x^2=w518:fxp<+,64,14>)
    n300 = Multiply(x=w516, y=w515) -> (x*y=w513:fxp<+/-,41,8>)
    "Sin omega_y" <- w513
    n301 = Negate(x=w518) -> (-x=w517:fxp<+/-,64,15>)
    n302 = Multiply(x=w513, y=w514) -> (x*y=w512:fxp<+/-,51,15>)
    n303 = Multiply(x=w517, y=w509) -> (x*y=w508:fxp<+/-,64,23>)
    n304 = Multiply(x=w511, y=w512) -> (x*y=→"Dyr_sin_d":fxp<+/-,64,16>)
    n305 = Multiply(x=w507, y=w508) -> (x*y=→"Dyr_sin_dd":fxp<+/-,64,25>)
    n306 = Multiply(x="Sin magnitude_y", y=w507) -> (x*y=w506:fxp<+/-,29,10>)
    n307 = Add(x=w506, y="Sin offset_y") -> (x+y=→"Dyr_sin":fxp<+/-,30,11>)
  }
  n308 = while "Encoder_y" {
    shift-right: [w563] -> _
    shift-left: _ -> [w561]
    shift-right: [w564] -> _
    shift-left: _ -> [w562]
    shift-right: [w567] -> _
    shift-left: _ -> [w566]
    stop <- FALSE stop-if-true
    n309 = xnode "FPGA I/O Node"() -> ("Mod4/DI0"=w568:bool, "Mod4/DI1"=w569:bool)  [unwired: 2 in, 2 out]
    n310 = call "encoder_sub.vi"("A_pre"=w561, "B_pre"=w562, "Encoder Position_pre"=w566, "A input"=w568, "Encoder Position Reset"="Encoder Reset_y", "B input"=w569) -> ("A"=w563:bool, "B"=w564:bool, "Encoder Position (Counts)"=w567:i32)  [unwired: 19 in]
    "Encoder Position_y" <- w567
    n311 = To Fixed-Point(number=w567) -> (fixed-point=w558:fxp<+/-,32,32>)  [unwired: 1 in]
    n312 = xnode "High Throughput Multiply"("x"=w558, "y"=fxp<+/-,24,0> 0.002499997615814209) -> ("x*y"=→"Dy (mm)":fxp<+/-,56,32>)
    n313 = xnode "High Throughput Multiply"("x"=w558, "y"=fxp<+/-,16,1> 0.125) -> ("x*y"=→"rad_y(NrTheta)":fxp<+/-,48,33>)
  }
  n314 = while "omega_y (M_avg)" {
    tunnel: w4 -> [w579]
    tunnel: w3 -> [w585]
    shift-right: [w575] -> _
    shift-left: w1 -> [w576]
    shift-right: [w574] -> _
    shift-left: w2 -> [w580]
    shift-right: [w572] -> _
    shift-left: _ -> [w577]
    stop <- FALSE stop-if-true
    w573 = fxp<+/-,27,3> 3.1415926218032837  # pi
    n315 = Multiply(x=w579, y=w585) -> (x*y=w584:u32)
    n316 = Index Array(array=w576, index=0) -> (element=w581:u32)
    n317 = Index Array(array=w580, index=0) -> (element=w578:i32)
    n318 = call "Tick Count5"() -> ("Tick Count(uSec)"=w582:u32)
    n319 = Add(x=w584, y=w581) -> (x+y=w588:u32)
    n320 = Greater Or Equal?(x=w582, y=w588) -> (x >= y?=w583:bool)
    n321 = case shown="True" w583 {
      tunnel: w582 -> [_ w611]
      tunnel: w581 -> [_ w612]
      tunnel: w580 -> [w590 w601]
      tunnel: w579 -> [_ w602]
      tunnel: w578 -> [_ w603]
      tunnel: w577 -> [w589 _]
      tunnel: w576 -> [w591 w613]
      tunnel: [w591 w594] -> w575
      tunnel: [w590 w593] -> w574
      tunnel: [w589 w592] -> w572
      frame False {
      }
      frame True {
        n322 = local read "Encoder Position_y"() -> (w604:i32)
        n323 = Subtract(x=w611, y=w612) -> (x-y=w610:u32)
        n324 = To Fixed-Point(number=w610) -> (fixed-point=w609:fxp<+,32,32>)  [unwired: 1 in]
        n325 = Subtract(x=w604, y=w603) -> (x-y=w605:i32)
        n326 = Multiply(x=w605, y=u32 2500) -> (x*y=w607:u32)
        n327 = Insert Into Array(array=w613, new element=w611) -> (w599:u32[])  [unwired: 1 in]
        n328 = Insert Into Array(array=w601, index=w602, new element=w604) -> (w600:i32[])
        n329 = To Fixed-Point(number=w607) -> (fixed-point=w608:fxp<+,32,32>)  [unwired: 1 in]
        n330 = Divide(x=w608, y=w609) -> (x/y=w592:fxp<+,64,32>)
        n331 = Delete From Array(array=w599, length=1, index=0) -> (array with subset deleted=w594:u32[])  [unwired: 1 out]
        n332 = Delete From Array(array=w600, length=1, index=0) -> (array with subset deleted=w593:i32[])  [unwired: 1 out]
      }
    }
    "Dy_d (M_avg)" <- w572
    n333 = Multiply(x=w573, y=w572) -> (x*y=→"omega_y(M_avg)":fxp<+/-,64,35>)
  }
  n334 = while "omega_y(M)" {
    shift-right: [w620] -> _
    shift-left: _ -> [w624]
    shift-right: [w621] -> _
    shift-left: _ -> [w623]
    shift-right: [w619] -> _
    shift-left: _ -> [w622]
    stop <- FALSE stop-if-true
    w616 = fxp<+/-,27,3> 3.1415926218032837  # pi
    n335 = local read "Encoder Position_y"() -> (w627:i32)
    n336 = call "Tick Count6"() -> ("Tick Count(mSec)"=w626:u32)
    n337 = call "M method (SubVI)_KY.vi"("Tc (mSec)"="Dy_d_M_Tc (mSec)", "Tick Count (mSec)"=w626, "Encoder velocity_pre (pulse/s)"=w622, "Shift Register in 2"=w623, "Shift Register in 1"=w624, "Encoder pulses"=w627) -> ("Encoder velocity (pulse/s)"=w619:fxp<+/-,64,32>, "Shift Register out 2"=w621:i32, "Shift Register out 1"=w620:u32)  [unwired: 3 in]
    n338 = Multiply(x=w619, y=fxp<+/-,20,-5> 0.002499997615814209) -> (x*y=w617:fxp<+/-,64,27>)
    "Dy_d (M)" <- w617
    n339 = Multiply(x=w616, y=w617) -> (x*y=→"omega_y (M)":fxp<+/-,64,30>)
  }
  n340 = while "omega_y (T)" {
    shift-right: [w638] -> _
    shift-left: _ -> [w637]
    shift-right: [w632] -> _
    shift-left: _ -> [w636]
    shift-right: [w639] -> _
    shift-left: _ -> [w635]
    stop <- FALSE stop-if-true
    n341 = local read "Encoder Position_y"() -> (w638:i32)
    n342 = call "Tick Count7"() -> ("Tick Count(Ticks)"=w634:u32)
    n343 = call "omega_sub_Encoder_800ppr.vi"("mt0"="mt0_y", "omega_pre"=w636, "ticks_m_pre"=w635, "ticks"=w634, "count_pre"=w637, "count"=w638) -> ("ticks_m"=w639:u32, "mt"=→"mt_y":u32, "omega"=w632:fxp<+/-,20,9>)  [unwired: 3 in]
    "omega_y (T)" <- w632
    n344 = xnode "High Throughput Multiply"("x"=fxp<+/-,26,1> 0.3183099031448364, "y"=w632) -> ("x*y"=→"Dy_d (T)":fxp<+/-,46,10>)
  }
  n345 = while "Velocity estiomation methods switch_y" {
    stop <- FALSE stop-if-true
    n346 = case shown="2" "Velocity Estimation_y" {
      tunnel: [w645 w646 w649] -> w642
      tunnel: [w644 w647 w648] -> w641
      frame 0, Default {
        n347 = local read "omega_y(M_avg)"() -> (w645:fxp<+/-,32,7>)
        n348 = local read "Dy_d (M_avg)"() -> (w644:fxp<+,32,8>)
      }
      frame 1 {
        n349 = local read "omega_y (M)"() -> (w646:fxp<+/-,32,7>)
        n350 = local read "Dy_d (M)"() -> (w647:fxp<+/-,32,8>)
      }
      frame 2 {
        n351 = local read "omega_y (T)"() -> (w649:fxp<+/-,32,7>)
        n352 = local read "Dy_d (T)"() -> (w648:fxp<+/-,32,8>)
      }
    }
    "omega_y (rad/s)" <- w642
    "Dy_d (mm/s)" <- w641
  }
  n353 = while "Integral and derivative_y" {
    shift-right: [w671] -> _
    shift-left: _ -> [w674]
    shift-right: [w660] -> _
    shift-left: _ -> [w651]
    shift-right: [w653] -> _
    shift-left: _ -> [w652]
    stop <- FALSE stop-if-true
    n354 = local read "Dy (mm)"() -> (w671:fxp<+/-,22,7>)
    n355 = local read "Dy_tolorence"() -> (w666:fxp<+/-,18,1>)
    n356 = local read "Dy_error"() -> (w663:fxp<+/-,24,8>)
    n357 = Subtract(x=w671, y=w674) -> (x-y=w673:fxp<+/-,23,8>)
    n358 = Absolute Value(x=w663) -> (abs(x)=w667:fxp<+,24,8>)
    n359 = Multiply(x=w673, y=fxp<+,7,10> 1000.0) -> (x*y=w670:fxp<+/-,30,18>)
    n360 = Greater?(x=w667, y=w666) -> (0:w665:bool)
    n361 = local read "Stop motor_y"() -> (w657:bool)
    n362 = Select(t=w663, s=w665, f=fxp<+,24,11> 0.0) -> (s? t:f=w660:fxp<+/-,28,12>)
    n363 = xnode "Butterworth Filter"("input data"=w670, "scaled coefficients"="scaled coefficients_Dy_dd") -> ("output data"=→"Dy_dd":fxp<+/-,34,22>)  [unwired: 1 in]
    n364 = Add(x=w651, y=w660) -> (x+y=w662:fxp<+/-,29,13>)
    n365 = Multiply(x=fxp<+/-,30,12> 0.000499725341796875, y=w662) -> (x*y=w659:fxp<+/-,58,24>)
    n366 = Select(t=fxp<+,1,1> 0.0, s=w657, f=fxp<+,1,1> 1.0) -> (s? t:f=w654:fxp<+,1,1>)
    n367 = Add(x=w659, y=w652) -> (x+y=w658:fxp<+/-,32,16>)
    n368 = Multiply(x=w658, y=w654) -> (x*y=w653:fxp<+/-,32,16>)
    "Dy_i" <- w653
    n369 = call "Wait4"("Count(uSec)"=u32 1000) -> ()  [unwired: 1 out]
  }
  n370 = while "Ramp gene._y" {
    stop <- FALSE stop-if-true
    n371 = flat-sequence {
      frame #0 {
        n372 = Divide(x="Dyr_end", y="Dyr_time") -> (x/y=→"Dyr_slope":fxp<+/-,64,30>)
      }
      frame #1 {
        n373 = local read "Time now_y (s)"() -> (w688:fxp<+,52,14>)
        n374 = while {
          tunnel: w688 -> [w693]
          stop <- FALSE stop-if-true
          n375 = local read "Time now_y (s)"() -> (w694:fxp<+,52,14>)
          n376 = local read "Dyr_slope"() -> (w691:fxp<+/-,32,10>)
          n377 = Subtract(x=w694, y=w693) -> (x-y=w692:fxp<+/-,53,15>)
          n378 = Multiply(x=w691, y=w692) -> (x*y=→"Dyr_ramp":fxp<+/-,64,24>)
        }
      }
    }
  }
